vi "Sequence Add.vi"(8 "error in (no error)":errorcluster, 10 "Sequence Record":T1, 11 "Connection Refnum":T2) -> (0 "error out":errorcluster, 2 "New Sequence Record":T1, 3 "Connection Refnum":T2)   [LabVIEW 2011]
uses:
  Sequence Record.ctl
  Summitek EXT/ODBC/SQL Controls/Connection Refnum.ctl
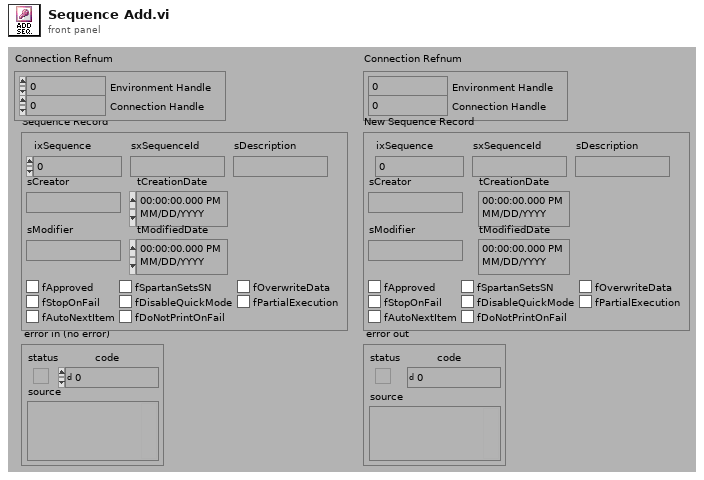
[diagram p1: front panel]
types:
  T1 = typedef "Sequence Record.ctl" = cluster{"ixSequence":i32, "sxSequenceId":string, "sDescription":string, "sCreator":string, "tCreationDate":timestamp, "sModifier":string, "tModifiedDate":timestamp, "fApproved":bool, "fSpartanSetsSN":bool, "fOverwriteData":bool, "fStopOnFail":bool, "fDisableQuickMode":bool, "fPartialExecution":bool, "fAutoNextItem":bool, "fDoNotPrintOnFail":bool}
  T2 = typedef "Connection Refnum.ctl" = cluster{"Environment Handle":i32, "Connection Handle":i32}
  T3 = typedef "Statement Refnum.ctl" = cluster{"Statement Handle":i32, "Parameter Number":u16}
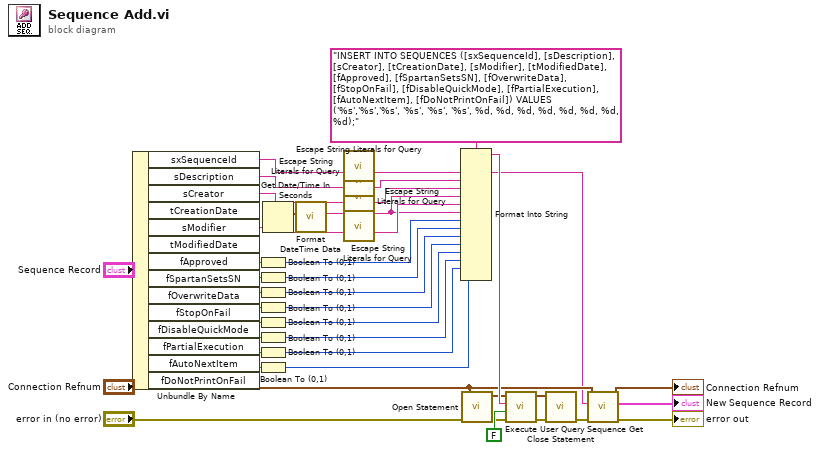
[diagram p0: block diagram]
diagram:
  n1 = Unbundle By Name("Sequence Record") -> ("sxSequenceId"=w30:string, "sDescription"=w29:string, "sCreator"=w27:string, "sModifier"=w21:string, "fApproved"=w20:bool, "fSpartanSetsSN"=w18:bool, "fOverwriteData"=w17:bool, "fStopOnFail"=w16:bool, "fDisableQuickMode"=w15:bool, "fPartialExecution"=w14:bool, "fAutoNextItem"=w13:bool, "fDoNotPrintOnFail"=w2:bool)  [unwired: 2 out]
  n2 = Boolean To (0,1)(Boolean=w20) -> (0, 1=w12:i16)
  n3 = Boolean To (0,1)(Boolean=w18) -> (0, 1=w11:i16)
  n4 = Boolean To (0,1)(Boolean=w17) -> (0, 1=w10:i16)
  n5 = Boolean To (0,1)(Boolean=w16) -> (0, 1=w9:i16)
  n6 = Boolean To (0,1)(Boolean=w15) -> (0, 1=w8:i16)
  n7 = Boolean To (0,1)(Boolean=w14) -> (0, 1=w7:i16)
  n8 = Boolean To (0,1)(Boolean=w13) -> (0, 1=w6:i16)
  n9 = Boolean To (0,1)(Boolean=w2) -> (0, 1=w1:i16)
  n10 = Get Date/Time In Seconds() -> (seconds since 1Jan1904=w3:timestamp)
  n11 = call "Format DateTime Data.vi"("Timestamp in"=w3) -> ("UTC DB String out"=w5:string)  [unwired: 10 out]
  n12 = call "Escape String Literals for Query.vi"("String"=w30) -> ("escaped String"=w4:string)  [unwired: 1 in, 13 out]
  n13 = call "Escape String Literals for Query.vi"("String"=w29) -> ("escaped String"=w28:string)  [unwired: 1 in, 13 out]
  n14 = call "Escape String Literals for Query.vi"("String"=w27) -> ("escaped String"=w26:string)  [unwired: 1 in, 13 out]
  n15 = call "Escape String Literals for Query.vi"("String"=w21) -> ("escaped String"=w19:string)  [unwired: 1 in, 13 out]
  n16 = Format Into String(format string="INSERT INTO SEQUENCES ([sxSequenceId], [sDescription], [sCreator], [tCreationDate], [sModifier], [tModifiedDate], [fApproved], [fSpartanSetsSN], [fOverwriteData], [fStopOnFail], [fDisableQuickMode], [fPartialExecution], [fAutoNextItem], [fDoNotPrintOnFail]) VALUES ('%s','%s','%s', '%s', '%s', '%s', %d, %d, %d, %d, %d, %d, %d, %d);" ("User Query"), w4, w28, w26, w5, w19, w5, w12, w11, w10, w9, w8, w7, w6, w1) -> (resulting string=w38:string)  [unwired: 2 in, 1 out]
  n17 = call "Open Statement.vi"("error in (no error)"="error in (no error)", "Connection Refnum"="Connection Refnum") -> ("error out"=w34:errorcluster, "Statement Refnum"=w33:T3)  [unwired: 4 out]
  n18 = call "Execute User Query.vi"("error in (no error)"=w34, "Return Data? (f)"=FALSE, "User Query"=w38, "Statement Refnum"=w33) -> ("error out"=w35:errorcluster, "Statement Refnum"=w36:T3)  [unwired: 2 out]
  n19 = call "Close Statement.vi"("error in (no error)"=w35, "Statement Refnum"=w36) -> ("error out"=w32:errorcluster)  [unwired: 5 out]
  n20 = call "Sequence Get.vi"("error in (no error)"=w32, "sxSequenceId (\"\")"=w4, "Connection Refnum"="Connection Refnum") -> ("error out"=→"error out":errorcluster, "Sequence Record"=→"New Sequence Record":T1, "Connection Refnum"=→"Connection Refnum":T2)  [unwired: 6 out]
